vi "LVTracker.vi"() -> ()   [LabVIEW 2011]
panel:
  in  "image in":u8[][](array[numeric])
  in  "input cluster":T1
  out "error in 2":errorcluster
  in  "error in":errorcluster
  out "LV tracker rad prof":dbl[](graph)
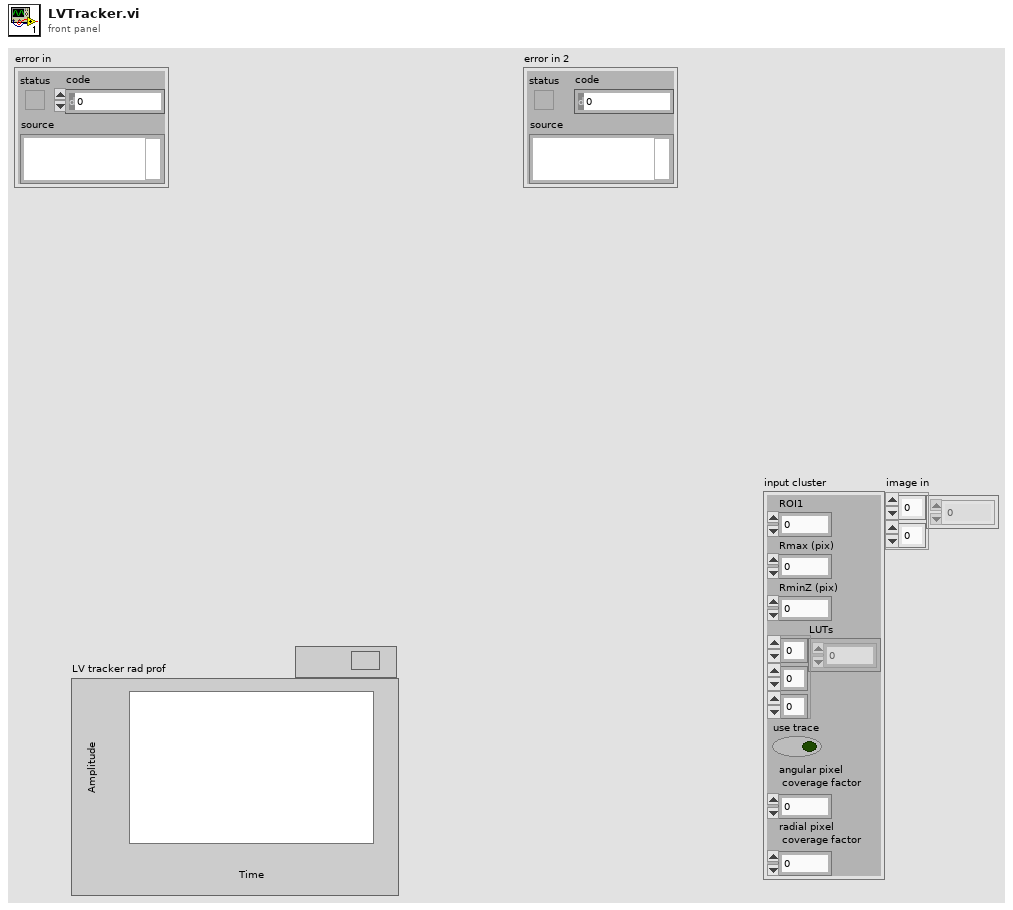
[diagram p1: front panel]
types:
  T1 = cluster{"ROI1":i32, "Rmax (pix)":i32, "RminZ (pix)":i32, "LUTs":dbl[][][], "use trace":bool, "angular pixel\n coverage factor":dbl, "radial pixel\n coverage factor":dbl}
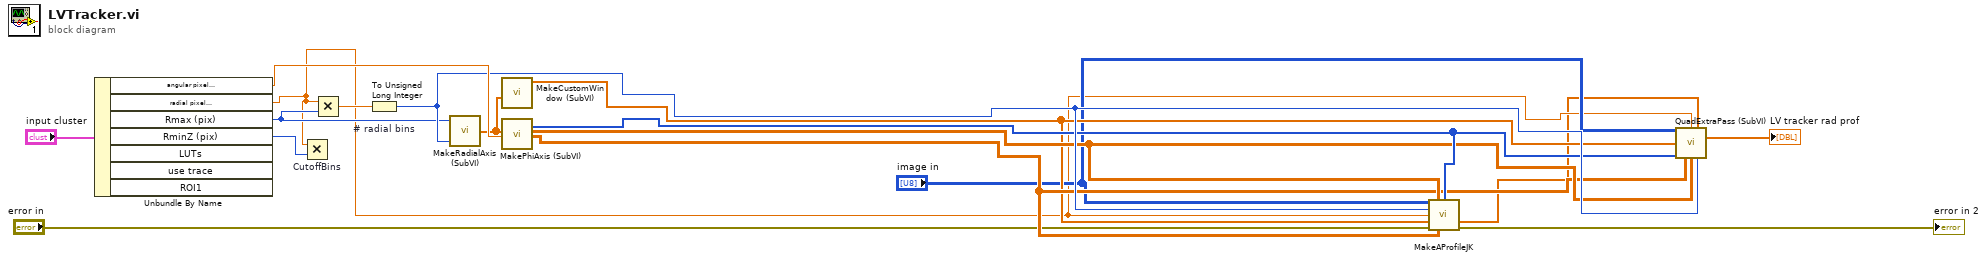
[diagram p0: block diagram]
diagram:
  n1 = Unbundle By Name("input cluster") -> ("angular pixel\n coverage factor"=w16:dbl, "radial pixel\n coverage factor"=w3:dbl, "Rmax (pix)"=w7:i32, "RminZ (pix)"=w9:i32)  [unwired: 3 out]
  n2 = Multiply "CutoffBins"(x=w3, y=w9) -> ()  [unwired: 1 out]
  n3 = Multiply(x=w3, y=w7) -> (x*y=w15:dbl)
  n4 = To Unsigned Long Integer "# radial bins"(number=w15) -> (unsigned 32bit integer=w13:u32)
  n5 = call "MakeRadialAxis (SubVI).vi"("# radial bins"=w13, "Rmax-Rmin"=w7) -> ("radialaxis"=w14:dbl[])  [unwired: 1 in]
  n6 = call "MakeCustomWindow (SubVI).vi"("radialaxis"=w14) -> ("Halfstetson"=w8:dbl[])  [unwired: 8 in, 2 out]
  n7 = call "MakePhiAxis (SubVI).vi"("radialBinAxis"=w14, "angular pixel \ncoverage factor"=w16) -> ("lengths"=w12:i32[], "Rsin(phi)[Q]"=w11:dbl[][][], "Rcos(phi)[Q]"=w10:dbl[][][])  [unwired: 2 in, 13 out]
  n8 = call "MakeAProfileJK.vi"("image in"="image in", "Rsin(phi)[Q]"=w11, "angularbinlengths"=w12, "# Radial bins"=w13, "radial bins/pixel"=w3, "window"=w8, "error in (no error) 2"="error in", "Rcos(phi)[Q]"=w10) -> ("xy-out 1"=w2:dbl[], "error in (no error) 3"=→"error in 2":errorcluster)  [unwired: 3 in, 3 out]
  n9 = call "QuadExtraPass (SubVI).vi"("Image"="image in", "radial bins/pixel"=w3, "First position"=w2, "window"=w8, "angularbinlengths"=w12, "Rcos(phi)[Q]"=w10, "Rsin(phi)[Q]"=w11, "# Radial bins"=w13) -> ("radial profile"=→"LV tracker rad prof":dbl[])  [unwired: 4 in, 3 out]
